vi "overlay gripper.vi"(10 "gripper":T1, 11 "Refnum in":T2) -> (3 "Refnum out":T2)   [LabVIEW 2018]
uses:
  <vilib>/vision/Image Controls.llb/IMAQ Image.ctl
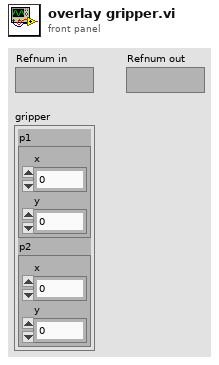
[diagram p1: front panel]
types:
  T1 = cluster{"p1":cluster{"x":dbl, "y":dbl}, "p2":cluster{"x":dbl, "y":dbl}}
  T2 = typedef "IMAQ Image.ctl" = refnum<image>
  T3 = cluster{"Desired Font (Application)":enum16{"User-specified Font", "Application Font", "System Font", "Dialog Font"}, "[User-specified Font]":cluster{"Font Name":string, "Size":i16, "Strikeout?":bool, "Italic?":bool, "Underline?":bool, "Outline?":bool, "Shadow?":bool, "Bold?":bool, "Rotation Angle":dbl}, "Horizontal Alignment":i16, "Vertical Alignment":i16}
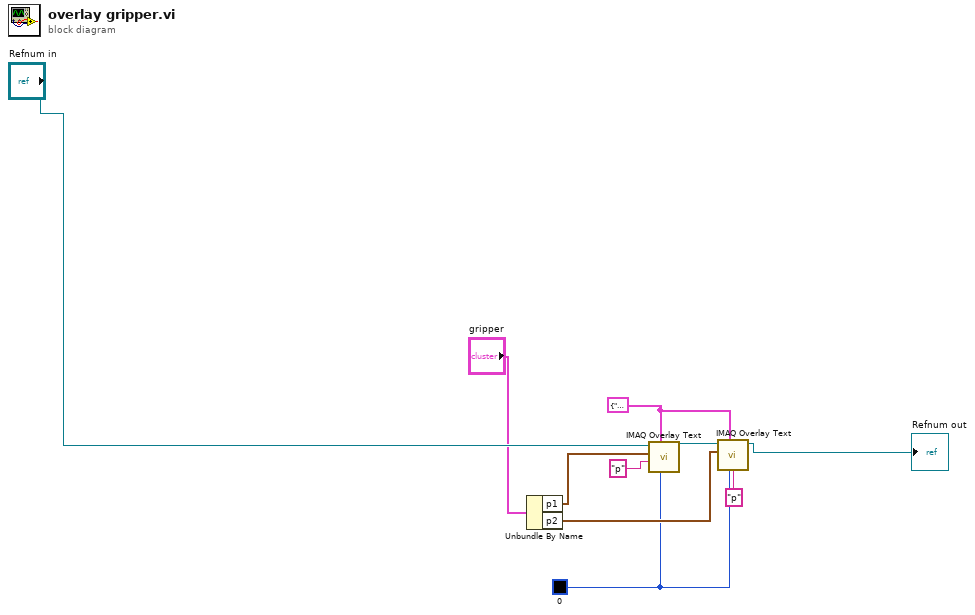
[diagram p0: block diagram]
diagram:
  w1 = u32 0 ("Text Color (black)")
  w2 = T3 {"Desired Font (Application)"=enum."User-specified Font", "[User-specified Font]"={"Font Name"="", "Size"=25, "Strikeout?"=FALSE, "Italic?"=FALSE, "Underline?"=TRUE, "Outline?"=FALSE, "Shadow?"=TRUE, "Bold?"=TRUE, "Rotation Angle"=0.0}, "Horizontal Alignment"=1, "Vertical Alignment"=2} ("Font, Size & Style")
  n1 = Unbundle By Name("gripper") -> ("p1"=w4:cluster{"x":dbl, "y":dbl}, "p2"=w9:cluster{"x":dbl, "y":dbl})
  n2 = call "IMAQ Overlay Text"("Text Color (black)"=w1, "Font, Size & Style"=w2, "String"="p", "Origin"=w4, "Image"="Refnum in") -> ("Image Out"=w8:T2)  [unwired: 5 in, 1 out]
  n3 = call "IMAQ Overlay Text"("Text Color (black)"=w1, "Font, Size & Style"=w2, "String"="p", "Origin"=w9, "Image"=w8) -> ("Image Out"=→"Refnum out":T2)  [unwired: 5 in, 1 out]
